vi "Table, Concatenate Row Headers.vi"(4 "error in":errorcluster, 6 "Tbl Refnum Dst":refnum<vi>, 7 "Tbl Refnum Src":refnum<vi>) -> (0 "error out":errorcluster, 2 "Tbl Refnum Dst out":refnum<vi>, 3 "Tbl Refnum Src out":refnum<vi>)   [LabVIEW 2010]
doc: "Copies the column headers (labels) of the source table to the destination table."
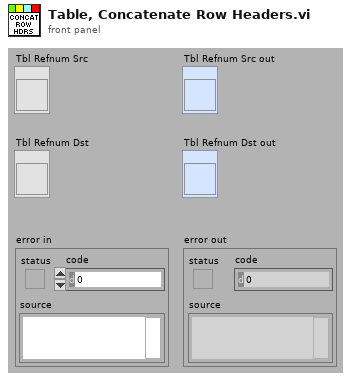
[diagram p1: front panel]
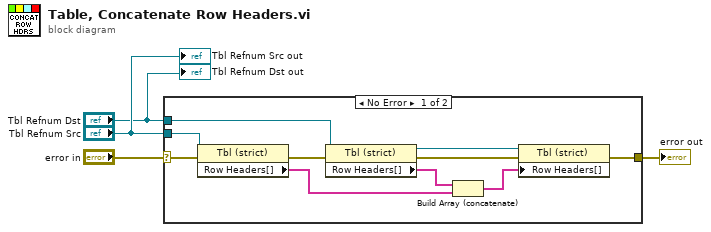
[diagram p0: block diagram]
diagram:
  n1 = case shown="No Error" "error in" {
    selector: "error in" -> [w12 w15]
    tunnel: [w13 w15] -> w4
    tunnel: "Tbl Refnum Dst" -> [w7 _]
    tunnel: "Tbl Refnum Src" -> [w8 _]
    frame No Error {
      n2 = property class="Tbl (strict)"(reference=w8, error in=w12) -> (error out=w11:errorcluster, "Row Headers[]"=w9:string[])  [unwired: 1 out]
      n3 = property class="Tbl (strict)"(reference=w7, error in=w11) -> (reference out=w6:refnum<vi>, error out=w14:errorcluster, "Row Headers[]"=w10:string[])
      n4 = Build Array (concatenate)(w10, w9) -> (w5:string[])
      n5 = property class="Tbl (strict)"(reference=w6, error in=w14, "Row Headers[]"=w5) -> (error out=w13:errorcluster)  [unwired: 1 out]
    }
    frame Error {
    }
  }
  "error out" <- w4
  "Tbl Refnum Src out" <- "Tbl Refnum Src"
  "Tbl Refnum Dst out" <- "Tbl Refnum Dst"
